vi "performZeroCalib.vi"(6 "Mode":i32(ring) items=["Current", "Charge", "Voltage", "Resistance"], 8 "error in (no error)":errorcluster, 9 "Input Range":dbl=10.0 format="%#_10g", 10 "Electrometer in":refnum<class "Electrometer.lvclass">, 11 "State in":refnum<class "State.lvclass">) -> (0 "error out":errorcluster, 1 "Range":string, 2 "Electrometer out":refnum<class "Electrometer.lvclass">, 3 "State out":refnum<class "State.lvclass">)   [LabVIEW 2016, in "State.lvclass"]
uses:
  State.lvclass
  Electrometer.lvclass
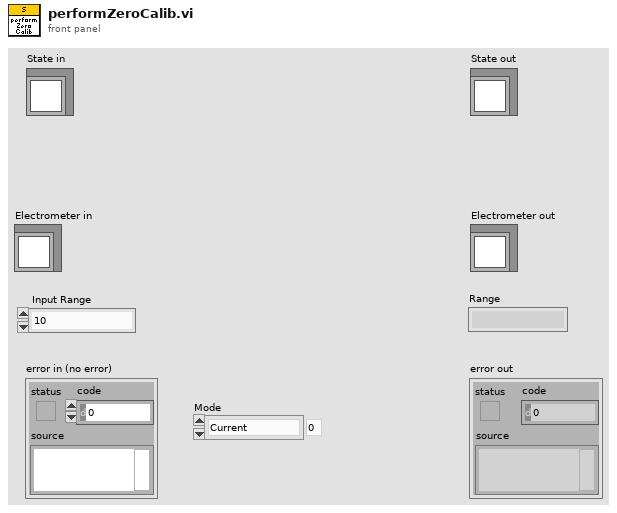
[diagram p1: front panel]
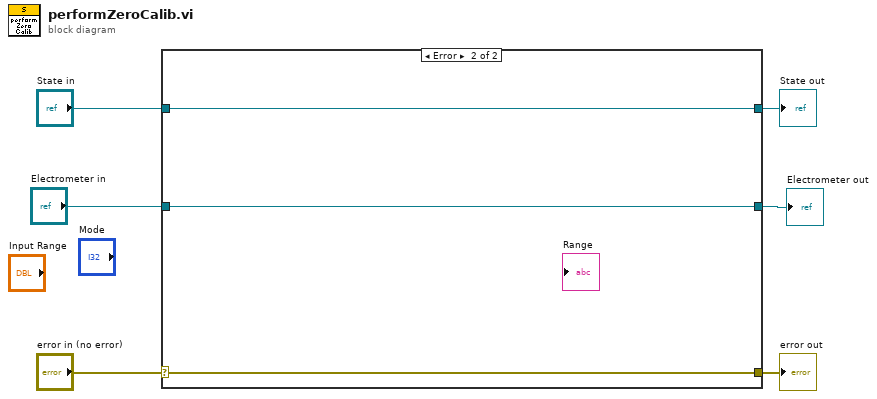
[diagram p0: block diagram]
diagram:
  n1 = case shown="Error" "error in (no error)" {
    selector: "error in (no error)" -> [w8 w12]
    tunnel: [w8 w12] -> w5
    tunnel: [w9 w11] -> w3
    tunnel: "State in" -> [w9 w11]
    tunnel: [w7 w10] -> w1
    tunnel: "Electrometer in" -> [w7 w10]
    frame No Error {
      # "Wire the error cluster across even in the \"No Error\"\ncase so that warnings get propagated."
    }
    frame Error {
    }
  }
  "error out" <- w5
  "State out" <- w3
  "Electrometer out" <- w1
